vi "HTTP Put.vi"(2 "Buffer":string, 3 "Endpoint":string="/SecondaryOutput/SetAttenuatorPercentage", 4 "Port":string="11200", 5 "IP Address":string="10.0.40.4") -> (0 "headers":string, 1 "body":string)   [LabVIEW 2020]
uses:
  <vilib>/httpClient/PUTBuffer.vi
  <vilib>/httpClient/LabVIEWHTTPClient.lvlib
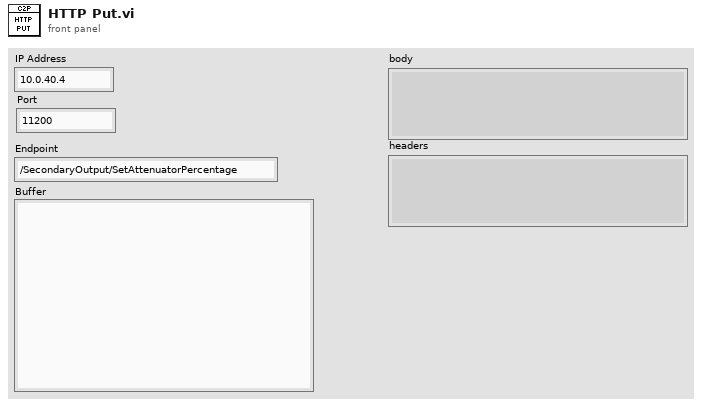
[diagram p1: front panel]
types:
  T1 = typedef "LabVIEWHTTPClient.lvlib/ClientHandle.ctl" = refnum<k1>
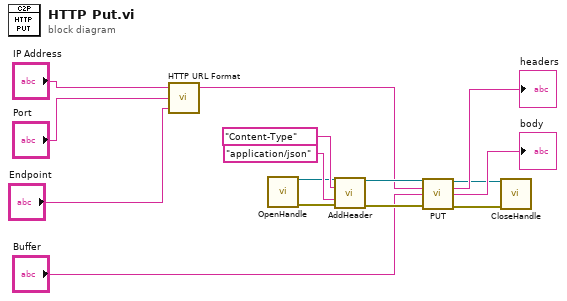
[diagram p0: block diagram]
diagram:
  n1 = call "HTTP URL Format.vi"("Endpoint"="Endpoint", "Port"="Port", "IP Address"="IP Address") -> ("URL"=w4:string)  [unwired: 2 in]
  n2 = call <vilib>:"OpenHandle.vi"() -> ("client handle out"=w8:T1, "error out"=w7:errorcluster)  [unwired: 14 in]
  n3 = call <vilib>:"AddHeader.vi"("client handle"=w8, "header"="Content-Type", "value"="application/json", "error in (no error)"=w7) -> ("client handle out"=w11:T1, "error out"=w10:errorcluster)  [unwired: 10 in]
  n4 = call-poly <vilib>:"PUT.vi"("client handle"=w11, "url"=w4, "buffer"="Buffer", "error in (no error)"=w10) -> ("client handle out"=w5:T1, "headers"=→"headers":string, "body"=→"body":string, "error out"=w6:errorcluster)  [unwired: 8 in]
  n5 = call <vilib>:"CloseHandle.vi"("client handle"=w5, "error in (no error)"=w6) -> ()  [unwired: 13 in, 1 out]
